vi "Initialize.vi"(8 "error in (no error)":errorcluster, 11 "Client in":refnum<class "Client.lvclass">) -> (0 "error out":errorcluster, 3 "Client out":refnum<class "Client.lvclass">)   [LabVIEW 2018, in "Client.lvclass"]
uses:
  Client.lvclass
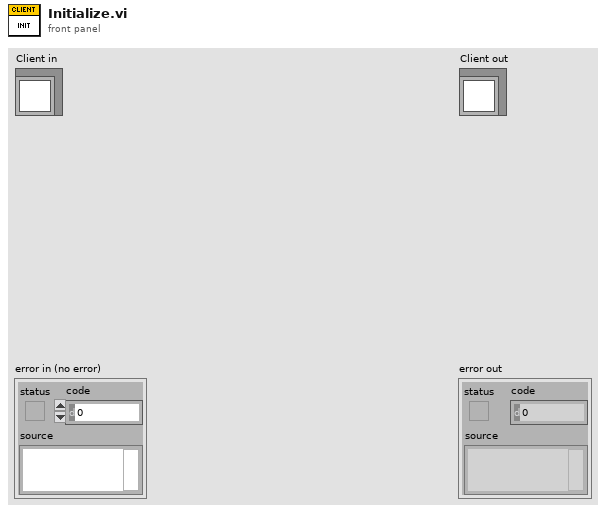
[diagram p1: front panel]
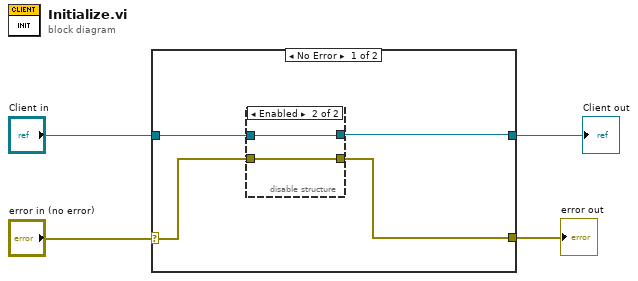
[diagram p0: block diagram]
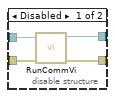
[diagram p2: hidden frame]
diagram:
  n1 = case shown="No Error" "error in (no error)" {
    selector: "error in (no error)" -> [w7 w16]
    tunnel: [w5 w16] -> w1
    tunnel: [w6 w15] -> w2
    tunnel: "Client in" -> [w8 w15]
    frame No Error {
      n2 = disable-structure shown="Enabled" {
        disable-tunnel: w8 -> [w12 w14]
        disable-tunnel: w7 -> [w11 w13]
        disable-tunnel: [w10 w14] -> w6
        disable-tunnel: [w9 w13] -> w5
        frame Disabled {
          n3 = call "RunCommVi.vi"("error in (no error)"=w11, "Client.lvclass in"=w12) -> ("error out"=w9:errorcluster, "Client.lvclass out"=w10:refnum<class "Client.lvclass">)  [unwired: 8 in]
        }
        frame Enabled {
        }
      }
    }
    frame Error {
    }
  }
  "error out" <- w1
  "Client out" <- w2
